vi "sub_EnableDisable Controls.vi"(8 "error in":errorcluster, 10 "Enable":bool, 11 "Controls":refnum<vi>[](array[refnum])) -> (0 "error out":errorcluster)   [LabVIEW 2012, in "PXImc System Explorer.lvlib"]
uses:
  PXImc System Explorer.lvlib
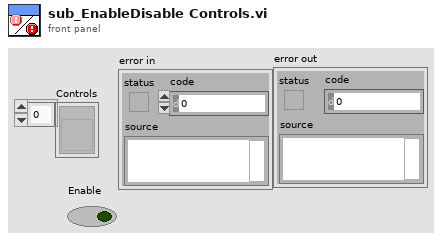
[diagram p1: front panel]
types:
  T1 = enum8{"Enabled", "Disabled", "Disabled and Grayed Out"}
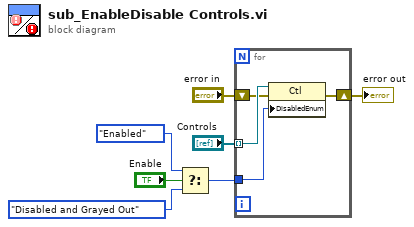
[diagram p0: block diagram]
diagram:
  n1 = Select(t=T1."Enabled" ("Disabled"), s="Enable", f=T1."Disabled and Grayed Out") -> (s? t:f=w4:T1)
  n2 = for {
    tunnel: "Controls" -> [w11] mode=indexing
    tunnel: w4 -> [w10]
    shift-right: [w8] -> w1
    shift-left: "error in" -> [w9]
    n3 = property class="Ctl"(reference=w11, error in=w9, "DisabledEnum"=w10) -> (error out=w8:errorcluster)  [unwired: 1 out]
  }
  "error out" <- w1
